vi "Operation Status (subVI).vi"(8 "Input Array":variant[](array[variant]), 11 "JSON string":string) -> (0 "output array":variant[](array[variant]))   [LabVIEW 2017]
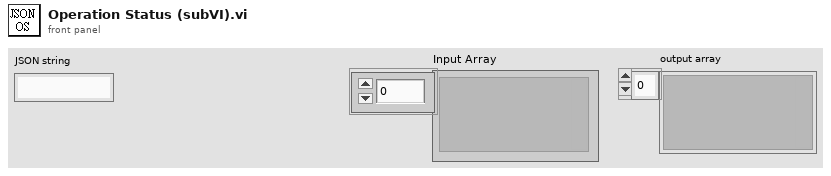
[diagram p1: front panel]
types:
  T1 = cluster{"ROperationStatus":string, "LOperationStatus":string}
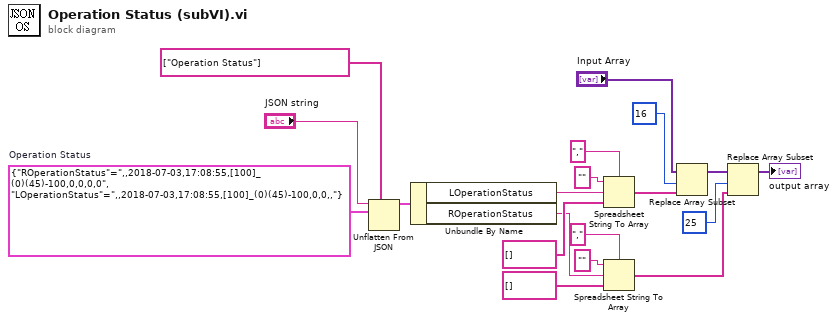
[diagram p0: block diagram]
diagram:
  w14 = T1 {"ROperationStatus"=",,2018-07-03,17:08:55,[100]_(0)(45)-100,0,0,0,0", "LOperationStatus"=",,2018-07-03,17:08:55,[100]_(0)(45)-100,0,0,,"}  # Operation Status
  n1 = Unflatten From JSON(path=string[] ["Operation Status"], JSON string="JSON string", type and defaults=w14) -> (value=w13:T1)  [unwired: 4 in, 1 out]
  n2 = Unbundle By Name(w13) -> ("LOperationStatus"=w12:string, "ROperationStatus"=w8:string)
  n3 = Spreadsheet String To Array(delimiter (Tab)=",", format string="", spreadsheet string=w12, array type (2D Dbl)=string[] []) -> (array=w5:string[])
  n4 = Spreadsheet String To Array(delimiter (Tab)=",", format string="", spreadsheet string=w8, array type (2D Dbl)=string[] []) -> (array=w3:string[])
  n5 = Replace Array Subset(array="Input Array", new element=w5, index=16) -> (w2:variant[])
  n6 = Replace Array Subset(array=w2, new element=w3, index=25) -> (→"output array":variant[])
